vi "Case Structure 3.vi"() -> ()   [LabVIEW 2020]
panel:
  out "Jumlah Iterasi":dbl
  out "Jumlah Klik":dbl
  in  "stop":bool
  out "Boolean 2":bool
  in  "BUTTON":bool
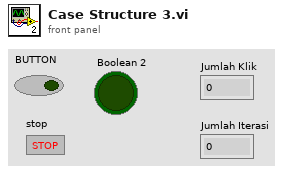
[diagram p1: front panel]
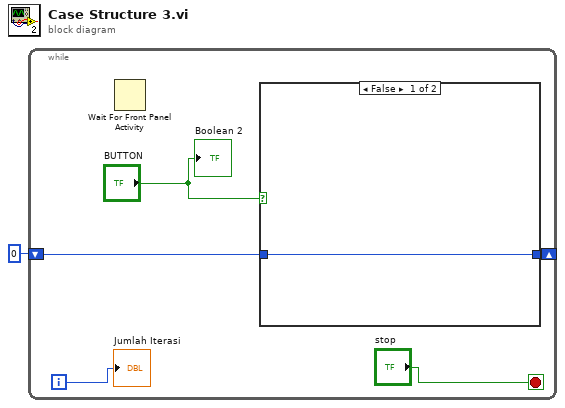
[diagram p0: block diagram]
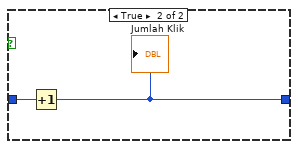
[diagram p2: hidden frame]
diagram:
  n1 = while {
    shift-right: [w3] -> _
    shift-left: 0 -> [w4]
    i -> [w2]
    stop <- "stop" stop-if-true
    n2 = Wait For Front Panel Activity() -> ()  [unwired: 3 in, 1 out]
    n3 = case shown="False" "BUTTON" {
      tunnel: w4 -> [w7 w9]
      tunnel: [w7 w8] -> w3
      frame False {
      }
      frame True {
        n4 = Increment(x=w9) -> (x+1=w8:i32)
        "Jumlah Klik" <- w8
      }
    }
    "Boolean 2" <- "BUTTON"
    "Jumlah Iterasi" <- w2
  }
